vi "WindDirectionInput.vi"() -> (3 "Wind Direction\n (Degrees)":dbl)   [LabVIEW 2016]
doc: "This VI is used to test the plausibility of the Wind Direction Sensor. \nIt gives the wind direction in degress.\n\nHere, input is an Analog signal in Voltage from MYRIO and outputs are Angle in degrees"
uses:
  <vilib>/myRIO/Instrument Drivers/Onboard IO/AI/typedefs/AI Reference.ctl
  <vilib>/myRIO/Common/Instrument Driver Framework/Utilities/typedefs/myRIO Generic Hardware Reference.ctl
  <vilib>/myRIO/Common/Instrument Driver Framework/Utilities/typedefs/Hardware Version Enum.ctl
  <vilib>/myRIO/Common/Instrument Driver Framework/Utilities/typedefs/myRIO v1.0 Reference.ctl
  <vilib>/myRIO/Common/Instrument Driver Framework/Utilities/typedefs/Generic FPGA Reference.ctl
  <vilib>/myRIO/Common/Instrument Driver Framework/myRIO v1.0/AI/typedefs/AI Channels List.ctl
  <vilib>/myRIO/Common/Instrument Driver Framework/myRIO v1.0/AI/typedefs/AI Channels Enum.ctl
  <vilib>/myRIO/Common/Instrument Driver Framework/Utilities/typedefs/Analog Scaling Constants List.ctl
  <vilib>/myRIO/Common/Instrument Driver Framework/Utilities/typedefs/Analog Scaling Constants.ctl
  <vilib>/userdefined/High Color/nirio_resource_hc.ctl
  <vilib>/myRIO/Common/Instrument Driver Framework/Utilities/vis/Is FPGA Ref Available.vi
  <vilib>/myRIO/Common/Instrument Driver Framework/myRIO v1.0/AI/vis/myRIO v1.1 Open AI.vi
  <vilib>/myRIO/Instrument Drivers/Onboard IO/AI/vis/Read.vi
  <vilib>/myRIO/Common/Instrument Driver Framework/Utilities/vis/Validate Channels.vi
  <vilib>/myRIO/Common/Instrument Driver Framework/myRIO v1.0/AI/vis/myRIO v1.0 Reserve AI.vi
  <vilib>/myRIO/Common/Instrument Driver Framework/myRIO v1.0/AI/vis/myRIO v1.0 Build MUX Configuration AI.vi
  <vilib>/myRIO/Common/Instrument Driver Framework/myRIO v1.0/Resource Manager/vis/myRIO v1.0 Reserve Channel List.vi
  <vilib>/myRIO/Common/Instrument Driver Framework/myRIO v1.0/Resource Manager/vis/myRIO v1.0 Reserve Channel.vi
  <vilib>/myRIO/Common/Instrument Driver Framework/myRIO v1.0/Resource Manager/vis/myRIO v1.0 Unreserve Channel.vi
  <vilib>/myRIO/Common/Instrument Driver Framework/myRIO v1.0/Resource Manager/vis/myRIO v1.0 Build Mutex Name.vi
  <vilib>/Utility/VariantDataType/GetNumericInfo.vi
  <vilib>/Utility/error.llb/Error Cluster From Error Code.vi
  <vilib>/myRIO/Common/Instrument Driver Framework/myRIO v1.0/myRIO v1.1 Open.vi
  <vilib>/myRIO/Common/Instrument Driver Framework/myRIO v1.0/AI/vis/myRIO v1.0 Get Scaling Constants AI.vi
  <vilib>/myRIO/Common/Instrument Driver Framework/Utilities/vis/IO Manager.vi
  <vilib>/myRIO/Common/Instrument Driver Framework/Utilities/vis/Configuration Manager.vi
  <vilib>/myRIO/Common/Instrument Driver Framework/myRIO v1.0/myRIO v1.0 Close.vi
  <vilib>/myRIO/Common/Instrument Driver Framework/myRIO v1.0/AI/vis/myRIO v1.0 Read AI.vi
  <vilib>/myRIO/Express VI/Onboard IO/AI/AI Express VI.xnode
  <vilib>/myRIO/Instrument Drivers/Onboard IO/AI/vis/myRIO AI Open.xnode
  <vilib>/myRIO/Instrument Drivers/Onboard IO/AI/AI.lvlib
panel:
  in  "stop":bool
  out "NNW":bool
  out "Input Signal in Voltage":dbl(graph)
  out "N":bool
  out "W":bool
  out "S":bool
  out "E":bool
  out "NW":bool
  out "SE":bool
  out "NE":bool
  out "WNW":bool
  out "WSW":bool
  out "SSW":bool
  out "ESE":bool
  out "NNE":bool
  out "SSE":bool
  out "SW":bool
  out "ENE":bool
  # "Here, we are assuming that, 0 degree denotes North and 180 degree denotes South"
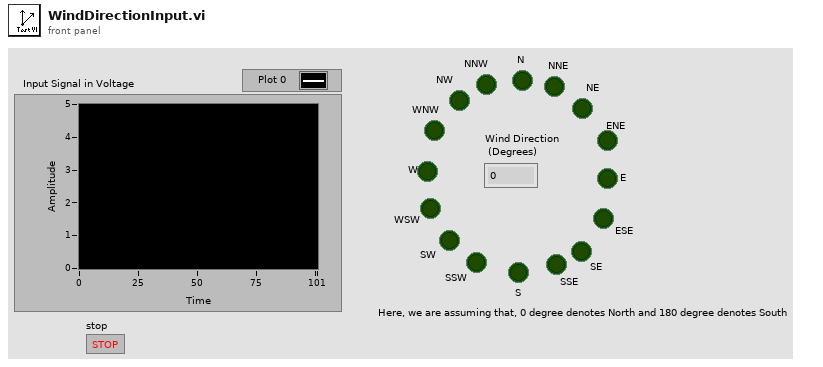
[diagram p1: front panel]
types:
  T1 = typedef "AI.lvlib/AI Reference.ctl" = cluster{"myRIO Reference":T2, "AI Channels List":T6, "AI Scaling Constants List":T8}
  T2 = typedef "myRIO Generic Hardware Reference.ctl" = cluster{"myRIO Model":T3, "myRIO Hardware Reference":T4}
  T3 = typedef "Hardware Version Enum.ctl" = enum16{"Unknown", "myRIO-1900", "myRIO-1950", "roboRIO", "NI ELVIS RIO CM"}
  T4 = typedef "myRIO v1.0 Reference.ctl" = cluster{"Generic FPGA Reference":T5, "Allow multiple opens":bool}
  T5 = typedef "Generic FPGA Reference.ctl" = refnum<k20>
  T6 = typedef "AI Channels List.ctl" = T7[]
  T7 = typedef "AI Channels Enum.ctl" = enum16{"Not Connected", "AudioIn/Left", "AudioIn/Right", "C/AI0", "C/AI1", "A/AI0", "A/AI1", "A/AI2", "A/AI3", "B/AI0", "B/AI1", "B/AI2", "B/AI3", "AI/AI0", "AI/AI1", "AI/AI2", "AI/AI3"}
  T8 = typedef "Analog Scaling Constants List.ctl" = T9[]
  T9 = typedef "Analog Scaling Constants.ctl" = cluster{"LSB Weight (Volts)":dbl, "Offset (Volts)":dbl, "Signed?":bool}
  T10 = typedef "nirio_resource_hc.ctl" = tag
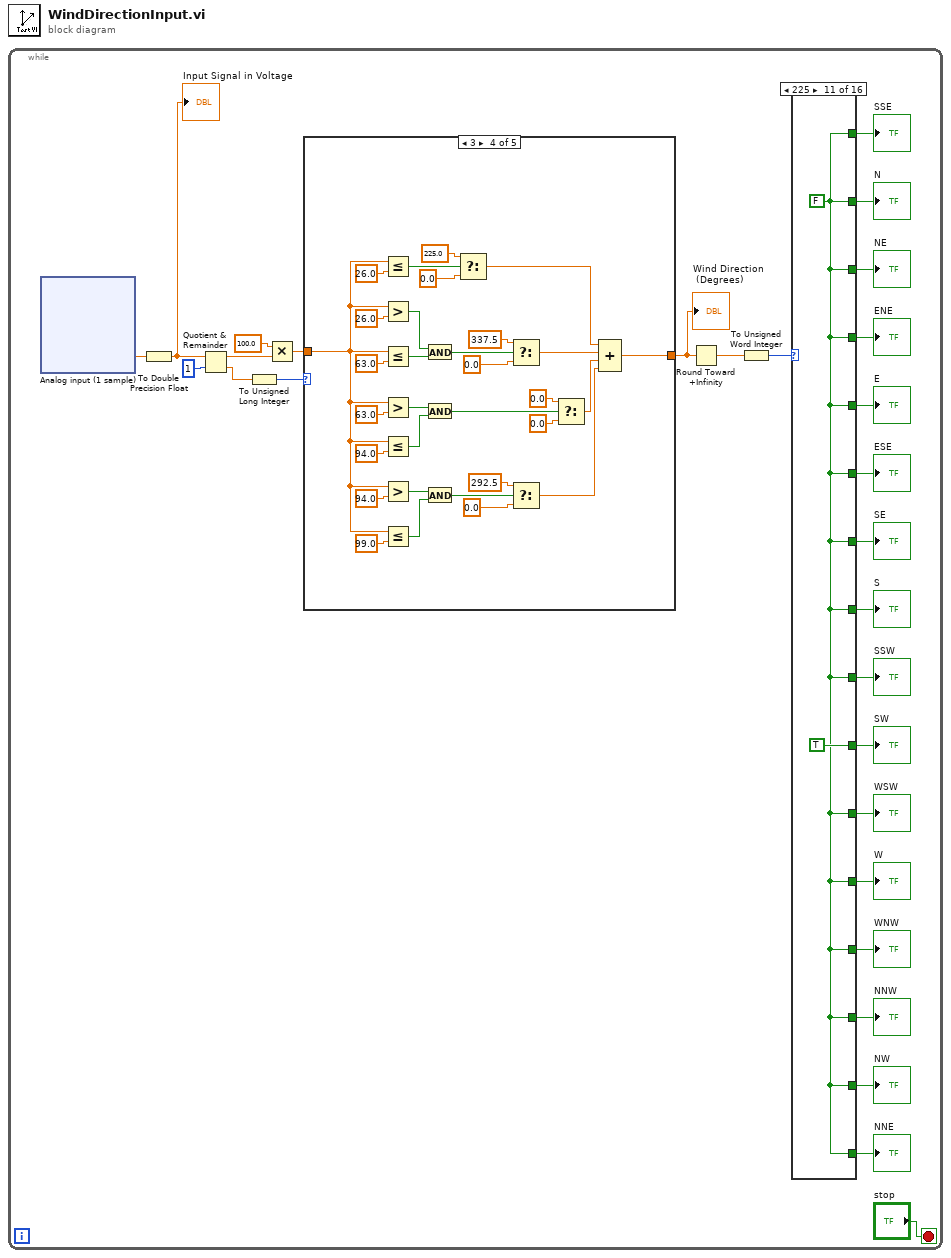
[diagram p0: block diagram]
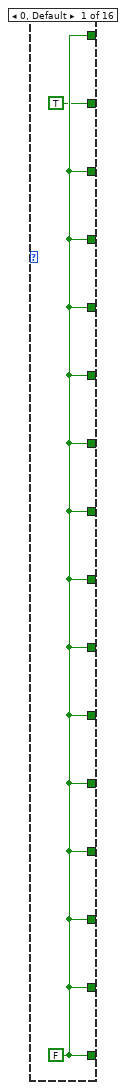
[diagram p2: hidden frame]
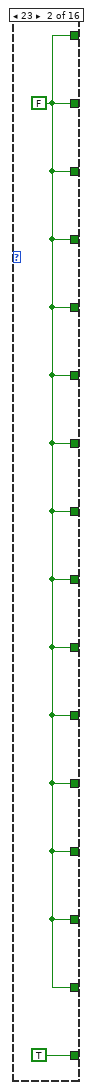
[diagram p3: hidden frame]
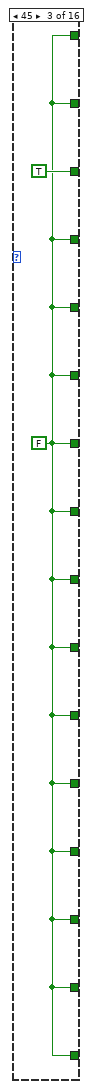
[diagram p4: hidden frame]
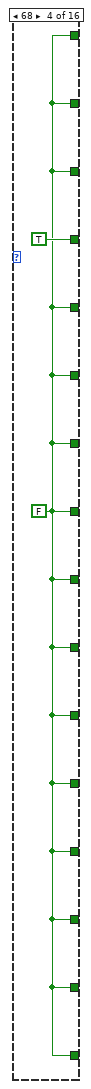
[diagram p5: hidden frame]
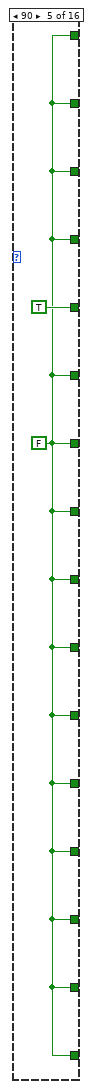
[diagram p6: hidden frame]
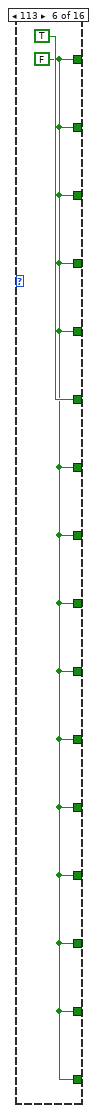
[diagram p7: hidden frame]
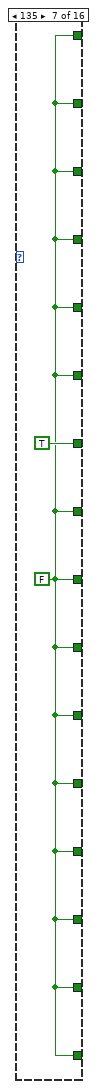
[diagram p8: hidden frame]
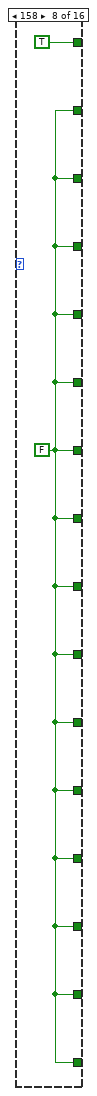
[diagram p9: hidden frame]
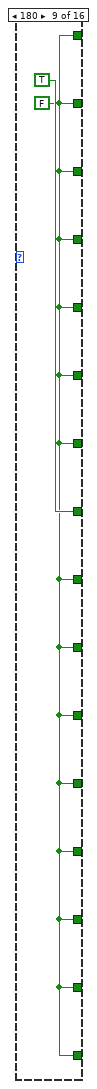
[diagram p10: hidden frame]
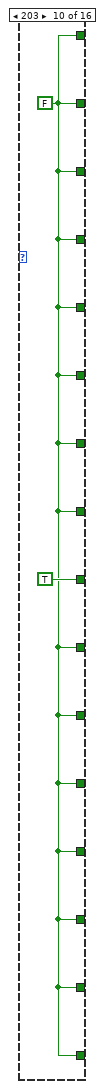
[diagram p11: hidden frame]
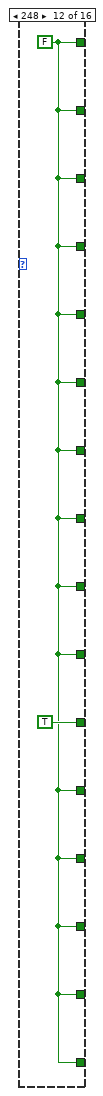
[diagram p12: hidden frame]
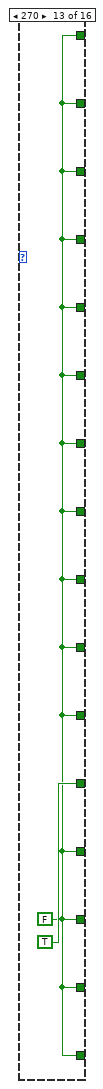
[diagram p13: hidden frame]
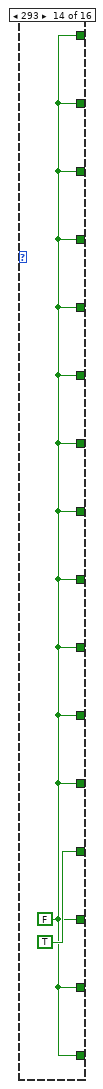
[diagram p14: hidden frame]
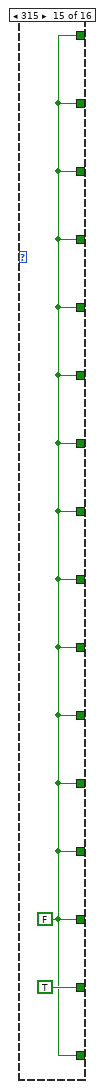
[diagram p15: hidden frame]
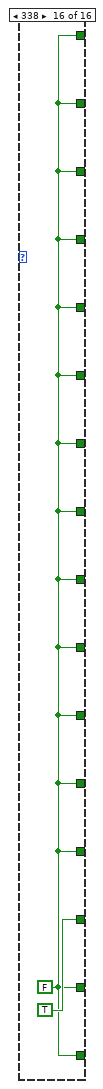
[diagram p16: hidden frame]
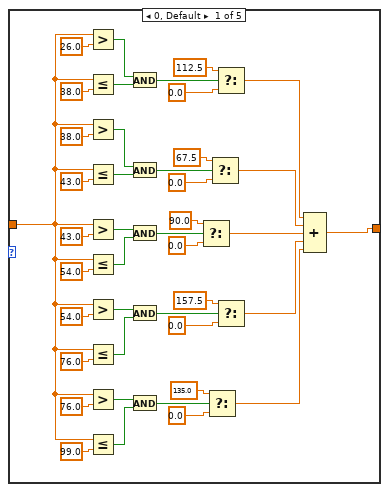
[diagram p17: hidden frame]
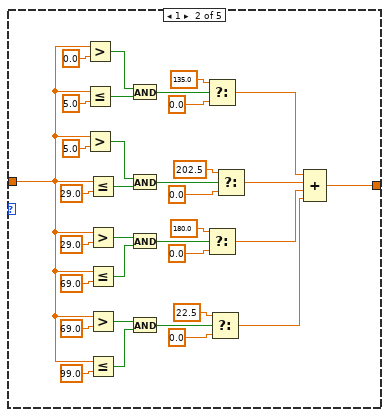
[diagram p18: hidden frame]
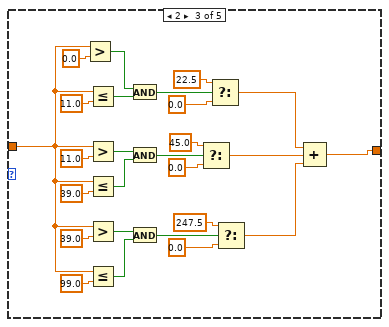
[diagram p19: hidden frame]
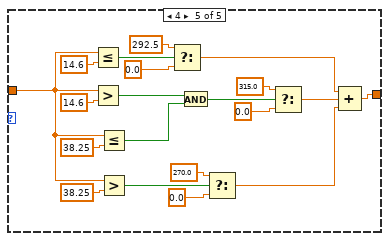
[diagram p20: hidden frame]
diagram:
  n1 = while {
    stop <- "stop" stop-if-true
    n2 = xnode "Analog input (1 sample)"() -> ("A/AI1 (Pin 5)"=w22:dbl)  [unwired: 1 in, 1 out]
    n3 = To Double Precision Float(number=w22) -> (double precision float=w21:dbl)
    "Input Signal in Voltage" <- w21
    n4 = Quotient & Remainder(x=w21, y=u8 1) -> (x-y*floor(x/y)=w24:dbl, floor(x/y)=w27:dbl)
    n5 = To Unsigned Long Integer(number=w27) -> (unsigned 32bit integer=w26:u32)
    n6 = Multiply(x=100.0, y=w24) -> (x*y=w23:dbl)
    n7 = case shown="3" w26 {
      tunnel: [w111 w159 w177 w219 w234] -> w2
      tunnel: w23 -> [w104 w145 w178 w206 w244]
      frame 0, Default {
        n8 = Greater?(x=w104, y=26.0) -> (0:w136:bool)
        n9 = Less Or Equal?(x=w104, y=38.0) -> (x <= y?=w137:bool)
        n10 = Greater?(x=w104, y=38.0) -> (0:w130:bool)
        n11 = Less Or Equal?(x=w104, y=43.0) -> (x <= y?=w131:bool)
        n12 = Greater?(x=w104, y=43.0) -> (0:w127:bool)
        n13 = Less Or Equal?(x=w104, y=54.0) -> (x <= y?=w128:bool)
        n14 = Greater?(x=w104, y=54.0) -> (0:w125:bool)
        n15 = Less Or Equal?(x=w104, y=76.0) -> (x <= y?=w124:bool)
        n16 = Greater?(x=w104, y=76.0) -> (0:w107:bool)
        n17 = Less Or Equal?(x=w104, y=99.0) -> (x <= y?=w108:bool)
        n18 = And(x=w136, y=w137) -> (x .and. y?=w102:bool)
        n19 = And(x=w130, y=w131) -> (x .and. y?=w101:bool)
        n20 = And(x=w127, y=w128) -> (x .and. y?=w100:bool)
        n21 = And(x=w125, y=w124) -> (x .and. y?=w99:bool)
        n22 = And(x=w107, y=w108) -> (x .and. y?=w98:bool)
        n23 = Select(t=90.0, s=w100, f=0.0) -> (s? t:f=w113:dbl)
        n24 = Select(t=135.0, s=w98, f=0.0) -> (s? t:f=w103:dbl)
        n25 = Select(t=67.5, s=w101, f=0.0) -> (s? t:f=w114:dbl)
        n26 = Select(t=112.5, s=w102, f=0.0) -> (s? t:f=w115:dbl)
        n27 = Select(t=157.5, s=w99, f=0.0) -> (s? t:f=w112:dbl)
        n28 = Compound Arithmetic op=ADD(w115, w114, w113, w112, w103) -> (w111:dbl)
      }
      frame 1 {
        n29 = Greater?(x=w145, y=0.0) -> (0:w146:bool)
        n30 = Less Or Equal?(x=w145, y=5.0) -> (x <= y?=w149:bool)
        n31 = Greater?(x=w145, y=5.0) -> (0:w173:bool)
        n32 = Less Or Equal?(x=w145, y=29.0) -> (x <= y?=w172:bool)
        n33 = Greater?(x=w145, y=29.0) -> (0:w166:bool)
        n34 = Less Or Equal?(x=w145, y=69.0) -> (x <= y?=w167:bool)
        n35 = Greater?(x=w145, y=69.0) -> (0:w156:bool)
        n36 = Less Or Equal?(x=w145, y=99.0) -> (x <= y?=w155:bool)
        n37 = And(x=w146, y=w149) -> (x .and. y?=w140:bool)
        n38 = And(x=w173, y=w172) -> (x .and. y?=w141:bool)
        n39 = And(x=w166, y=w167) -> (x .and. y?=w142:bool)
        n40 = And(x=w156, y=w155) -> (x .and. y?=w143:bool)
        n41 = Select(t=135.0, s=w140, f=0.0) -> (s? t:f=w144:dbl)
        n42 = Select(t=180.0, s=w142, f=0.0) -> (s? t:f=w160:dbl)
        n43 = Select(t=22.5, s=w143, f=0.0) -> (s? t:f=w152:dbl)
        n44 = Select(t=202.5, s=w141, f=0.0) -> (s? t:f=w161:dbl)
        n45 = Compound Arithmetic op=ADD(w144, w161, w160, w152) -> (w159:dbl)
      }
      frame 2 {
        n46 = Greater?(x=w178, y=0.0) -> (0:w197:bool)
        n47 = Less Or Equal?(x=w178, y=11.0) -> (x <= y?=w196:bool)
        n48 = Greater?(x=w178, y=11.0) -> (0:w191:bool)
        n49 = Less Or Equal?(x=w178, y=39.0) -> (x <= y?=w190:bool)
        n50 = Greater?(x=w178, y=39.0) -> (0:w184:bool)
        n51 = Less Or Equal?(x=w178, y=99.0) -> (x <= y?=w185:bool)
        n52 = And(x=w197, y=w196) -> (x .and. y?=w175:bool)
        n53 = And(x=w191, y=w190) -> (x .and. y?=w176:bool)
        n54 = And(x=w184, y=w185) -> (x .and. y?=w174:bool)
        n55 = Select(t=45.0, s=w176, f=0.0) -> (s? t:f=w180:dbl)
        n56 = Select(t=22.5, s=w175, f=0.0) -> (s? t:f=w181:dbl)
        n57 = Select(t=247.5, s=w174, f=0.0) -> (s? t:f=w179:dbl)
        n58 = Compound Arithmetic op=ADD(w181, w180, w179) -> (w177:dbl)
      }
      frame 3 {
        n59 = Less Or Equal?(x=w206, y=26.0) -> (x <= y?=w203:bool)
        n60 = Greater?(x=w206, y=26.0) -> (0:w229:bool)
        n61 = Less Or Equal?(x=w206, y=63.0) -> (x <= y?=w228:bool)
        n62 = Greater?(x=w206, y=63.0) -> (0:w213:bool)
        n63 = Less Or Equal?(x=w206, y=94.0) -> (x <= y?=w214:bool)
        n64 = Greater?(x=w206, y=94.0) -> (0:w212:bool)
        n65 = Less Or Equal?(x=w206, y=99.0) -> (x <= y?=w211:bool)
        n66 = And(x=w229, y=w228) -> (x .and. y?=w202:bool)
        n67 = And(x=w213, y=w214) -> (x .and. y?=w201:bool)
        n68 = And(x=w212, y=w211) -> (x .and. y?=w200:bool)
        n69 = Select(t=225.0, s=w203, f=0.0) -> (s? t:f=w221:dbl)
        n70 = Select(t=337.5, s=w202, f=0.0) -> (s? t:f=w220:dbl)
        n71 = Select(t=292.5, s=w200, f=0.0) -> (s? t:f=w204:dbl)
        n72 = Select(t=0.0, s=w201, f=0.0) -> (s? t:f=w205:dbl)
        n73 = Compound Arithmetic op=ADD(w221, w220, w205, w204) -> (w219:dbl)
      }
      frame 4 {
        n74 = Less Or Equal?(x=w244, y=14.6) -> (x <= y?=w233:bool)
        n75 = Greater?(x=w244, y=14.6) -> (0:w250:bool)
        n76 = Less Or Equal?(x=w244, y=38.25) -> (x <= y?=w249:bool)
        n77 = Greater?(x=w244, y=38.25) -> (0:w231:bool)
        n78 = Select(t=292.5, s=w233, f=0.0) -> (s? t:f=w237:dbl)
        n79 = And(x=w250, y=w249) -> (x .and. y?=w232:bool)
        n80 = Select(t=270.0, s=w231, f=0.0) -> (s? t:f=w235:dbl)
        n81 = Select(t=315.0, s=w232, f=0.0) -> (s? t:f=w236:dbl)
        n82 = Compound Arithmetic op=ADD(w237, w236, w235) -> (w234:dbl)
      }
    }
    "Wind Direction\n (Degrees)" <- w2
    n83 = Round Toward +Infinity(x=w2) -> (ceil(x): smallest int >= x=w1:dbl)
    n84 = To Unsigned Word Integer(number=w1) -> (unsigned 16bit integer=w20:u16)
    n85 = case shown="225" w20 {
      tunnel: [w30 TRUE w33 w35 w37 w39 w41 w43 w45 w47 w49 w51 w53 w55 w57 w59] -> w19
      tunnel: [w30 w31 TRUE w35 w37 w39 w41 w43 w45 w47 w49 w51 w53 w55 w57 w59] -> w18
      tunnel: [w30 w31 w33 TRUE w37 w39 w41 w43 w45 w47 w49 w51 w53 w55 w57 w59] -> w17
      tunnel: [w30 w31 w33 w35 TRUE w39 w41 w43 w45 w47 w49 w51 w53 w55 w57 w59] -> w16
      tunnel: [w30 w31 w33 w35 w37 TRUE w41 w43 w45 w47 w49 w51 w53 w55 w57 w59] -> w15
      tunnel: [w30 w31 w33 w35 w37 w39 TRUE w43 w45 w47 w49 w51 w53 w55 w57 w59] -> w14
      tunnel: [w30 w31 w33 w35 w37 w39 w41 TRUE w45 w47 w49 w51 w53 w55 w57 w59] -> w13
      tunnel: [w30 w31 w33 w35 w37 w39 w41 w43 TRUE w47 w49 w51 w53 w55 w57 w59] -> w12
      tunnel: [w30 w31 w33 w35 w37 w39 w41 w43 w45 TRUE w49 w51 w53 w55 w57 w59] -> w11
      tunnel: [w30 w31 w33 w35 w37 w39 w41 w43 w45 w47 TRUE w51 w53 w55 w57 w59] -> w10
      tunnel: [w30 w31 w33 w35 w37 w39 w41 w43 w45 w47 w49 TRUE w53 w55 w57 w59] -> w9
      tunnel: [w30 w31 w33 w35 w37 w39 w41 w43 w45 w47 w49 w51 TRUE w55 w57 w59] -> w8
      tunnel: [w30 w31 w33 w35 w37 w39 w41 w43 w45 w47 w49 w51 w53 TRUE w57 w59] -> w7
      tunnel: [w30 w31 w33 w35 w37 w39 w41 w43 w45 w47 w49 w51 w53 w55 TRUE w59] -> w6
      tunnel: [w30 w31 w33 w35 w37 w39 w41 w43 w45 w47 w49 w51 w53 w55 w57 TRUE] -> w5
      tunnel: [TRUE w31 w33 w35 w37 w39 w41 w43 w45 w47 w49 w51 w53 w55 w57 w59] -> w4
      frame 0, Default {
        w30 = FALSE
      }
      frame 23 {
        w31 = FALSE
      }
      frame 45 {
        w33 = FALSE
      }
      frame 68 {
        w35 = FALSE
      }
      frame 90 {
        w37 = FALSE
      }
      frame 113 {
        w39 = FALSE
      }
      frame 135 {
        w41 = FALSE
      }
      frame 158 {
        w43 = FALSE
      }
      frame 180 {
        w45 = FALSE
      }
      frame 203 {
        w47 = FALSE
      }
      frame 225 {
        w49 = FALSE
      }
      frame 248 {
        w51 = FALSE
      }
      frame 270 {
        w53 = FALSE
      }
      frame 293 {
        w55 = FALSE
      }
      frame 315 {
        w57 = FALSE
      }
      frame 338 {
        w59 = FALSE
      }
    }
    "WSW" <- w9
    "W" <- w8
    "WNW" <- w7
    "N" <- w4
    "NNE" <- w19
    "NE" <- w18
    "ENE" <- w17
    "E" <- w16
    "ESE" <- w15
    "SE" <- w14
    "SSE" <- w13
    "S" <- w12
    "SSW" <- w11
    "SW" <- w10
    "NW" <- w6
    "NNW" <- w5
  }
